vi "ConvertToFXP.vi"(11 "TotalTime":u32) -> (3 "x/y":fxp<+,64,32> format="%#_6p")   [LabVIEW 2019]
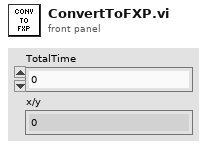
[diagram p1: front panel]
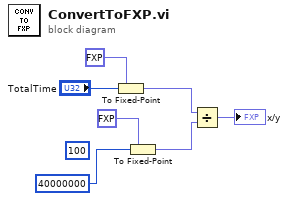
[diagram p0: block diagram]
diagram:
  (unwired) u32 100 ("y")
  n1 = To Fixed-Point(fixed-point type=fxp<+,32,32> 0.0, number="TotalTime") -> (fixed-point=w4:fxp<+,32,32>)
  n2 = To Fixed-Point(fixed-point type=fxp<+,32,32> 0.0, number=u32 40000000 ("y")) -> (fixed-point=w3:fxp<+,32,32>)
  n3 = Divide(x=w4, y=w3) -> (x/y=→"x/y":fxp<+,64,32>)
